vi "AIT 664 - Create Hardware Output Channels Tx Ports.vi"(0 "Device Reference in":T8 format="%.0x", 5 "End System Handle in":u64, 7 "End System References In":T8[](array[typedef]) format="%.0x", 9 "FIFO Index Queues":T13, 11 "error in (no error)":errorcluster) -> (3 "Hardware Output - Tx Ports":T1[](array[typedef]) {"Message Settings"."Transmit Channel Data Reference" format="%.0x"; "Message Settings"."Queue Transmit Channel" format="%.0x"; "Message Settings"."Driver Data"."Num Bits" min=1 max=32; "Message Settings"."Block Data Refs"."Data Reference" format="%.0x"; "Rx Com Udp Port"."Handle" format="%08x"; "Tx Com Udp Port"."Handle" format="%08x"}, 15 "error out":errorcluster)   [LabVIEW 2013, in "AIT 664 Custom Device.lvlib"]
doc: "For each Output VL page, find all of the Tx Mesage Ports Pages and configure the AIT 664 ComUdp port and all of the channels defined by the user for that port.\n\nReturns configured hardware channels and open AIT 664 Com Udp Port."
uses:
  AIT 664 Custom Device.lvlib
  <vilib>/NI Veristand/Custom Device API/Custom Device Item Ref.ctl
  RT Controls/FIFO Index Queues.ctl
  RT Controls/AIT 664 - RT Hardware Channel.ctl
  RT Controls/AIT 664 - RT Message Settings.ctl
  <vilib>/NI Veristand/Custom Device API/Block Data Reference.ctl
  <vilib>/NI Veristand/Custom Device API/Data Reference.ctl
  RT Controls/AIT 664 - Driver Data.ctl
  Controls and Global/Start Bit.ctl
  Controls and Global/Number of Bits.ctl
  <userlib>/ARINC 664/AIT 664 Controls/General/Message Port.ctl
  <userlib>/ARINC 664/AIT 664 Controls/General/Direction.ctl
  <userlib>/ARINC 664/AIT 664 Controls/General/Message Port Type.ctl
  System Explorer/Controls/664 - Sampling Type.ctl
  <vilib>/NI Veristand/Custom Device API/Data Access Type.ctl
  <vilib>/NI Veristand/Custom Device Tools/Custom Device Utility Library/NI VeriStand - Search for All Items by GUID.vi
  Controls and Global/Global.vi
  <vilib>/NI Veristand/Custom Device API/Get Item Property (U32).vi
  <vilib>/NI Veristand/Custom Device API/Get Item Property (Variant).vi
  <instrlib>/AIT 664/Private/AIT 664 Configure/Tx/Open/AIT 664 Tx Open Message Port (ComUdp).vi
  <userlib>/ARINC 664/AIT 664 API.lvlib
  <vilib>/NI Veristand/Custom Device API/Custom Device API.lvlib
  <vilib>/NI Veristand/Custom Device Tools/Custom Device Utility Library/Custom Device Utility Library.lvlib
  <instrlib>/AIT 664/AIT 664.lvlib
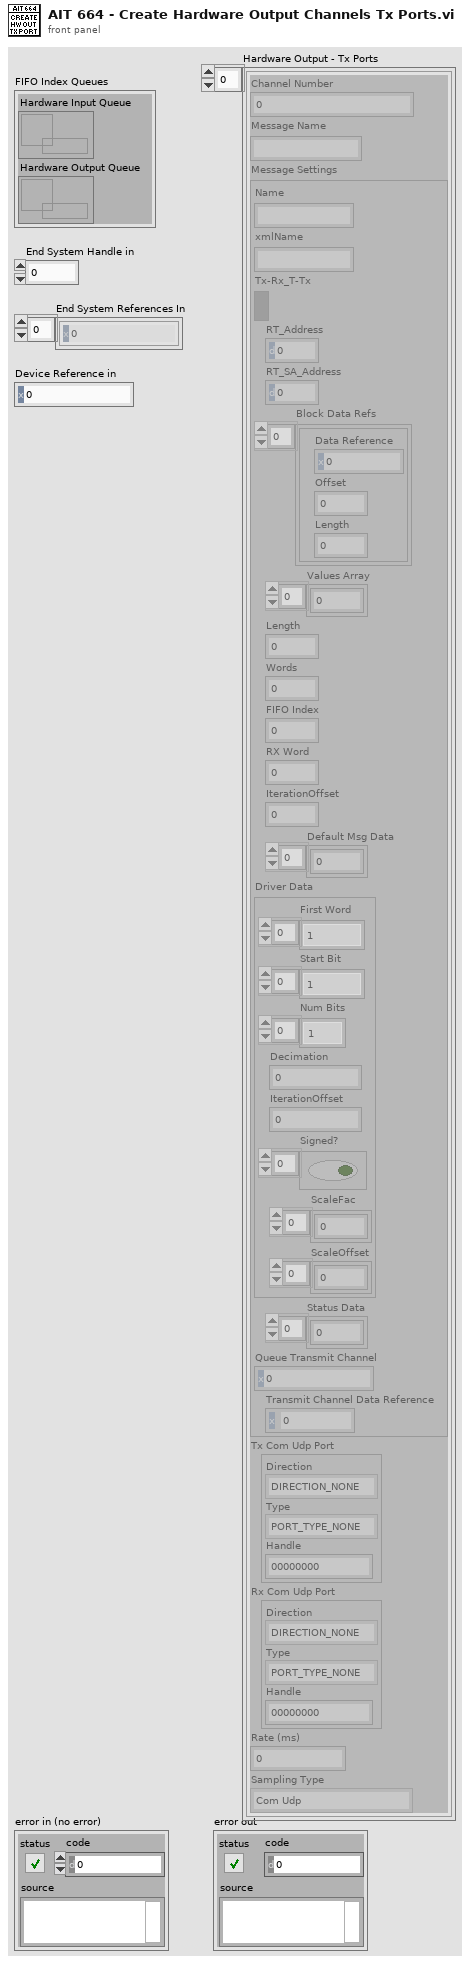
[diagram p1: front panel]
types:
  T1 = typedef "AIT 664 Custom Device.lvlib/AIT 664 - RT Hardware Channel.ctl" = cluster{"Channel Number":u16, "Message Name":string, "Message Settings":T2, "Tx Com Udp Port":T9, "Rx Com Udp Port":T9, "Rate (ms)":u32, "Sampling Type":T12}
  T2 = typedef "AIT 664 Custom Device.lvlib/AIT 664 - RT Message Settings.ctl" = cluster{"Name":string, "xmlName":string, "Tx-Rx_T-Tx":bool, "RT_Address":u8, "RT_SA_Address":u8, "Block Data Refs":T3[], "Values Array":dbl[], "Length":i32, "Words":i32, "FIFO Index":i32, "RX Word":u32, "IterationOffset":i32, "Default Msg Data":u8[], "Driver Data":T5, "Status Data":u32[], "Queue Transmit Channel":T8, "Transmit Channel Data Reference":T4}
  T3 = typedef "Custom Device API.lvlib/Block Data Reference.ctl" = cluster{"Data Reference":T4, "Offset":i32, "Length":i32}
  T4 = typedef "Custom Device API.lvlib/Data Reference.ctl" = i32
  T5 = typedef "AIT 664 Custom Device.lvlib/AIT 664 - Driver Data.ctl" = cluster{"First Word":T6[], "Start Bit":T6[], "Num Bits":T7[], "Decimation":i32, "IterationOffset":i32, "Signed?":bool[], "ScaleFac":dbl[], "ScaleOffset":dbl[]}
  T6 = typedef "AIT 664 Custom Device.lvlib/Start Bit.ctl" = i32
  T7 = typedef "AIT 664 Custom Device.lvlib/Number of Bits.ctl" = i32
  T8 = typedef "Custom Device API.lvlib/Custom Device Item Ref.ctl" = u64
  T9 = typedef "AIT 664 API.lvlib/Message Port.ctl" = cluster{"Direction":T10, "Type":T11, "Handle":u64}
  T10 = typedef "AIT 664 API.lvlib/Direction.ctl" = enum16{"DIRECTION_NONE", "DIRECTION_TX", "DIRECTION_RX"}
  T11 = typedef "AIT 664 API.lvlib/Message Port Type.ctl" = enum16{"PORT_TYPE_NONE", "COM_UDP", "SAP_UDP", "SAP_IP", "SAP_MAC", "COTS_MAC", "COTS_MAC_RAW"}
  T12 = typedef "AIT 664 Custom Device.lvlib/664 - Sampling Type.ctl" = enum16{"Com Udp", "Com Udp Queuing", "Sap Udp", "Sap Ip", "Sap Mac", "Unknown"}
  T13 = typedef "AIT 664 Custom Device.lvlib/FIFO Index Queues.ctl" = cluster{"Hardware Input Queue":refnum<queue>, "Hardware Output Queue":refnum<queue>}
  T14 = typedef "Custom Device API.lvlib/Data Access Type.ctl" = enum16{"Read", "Write"}
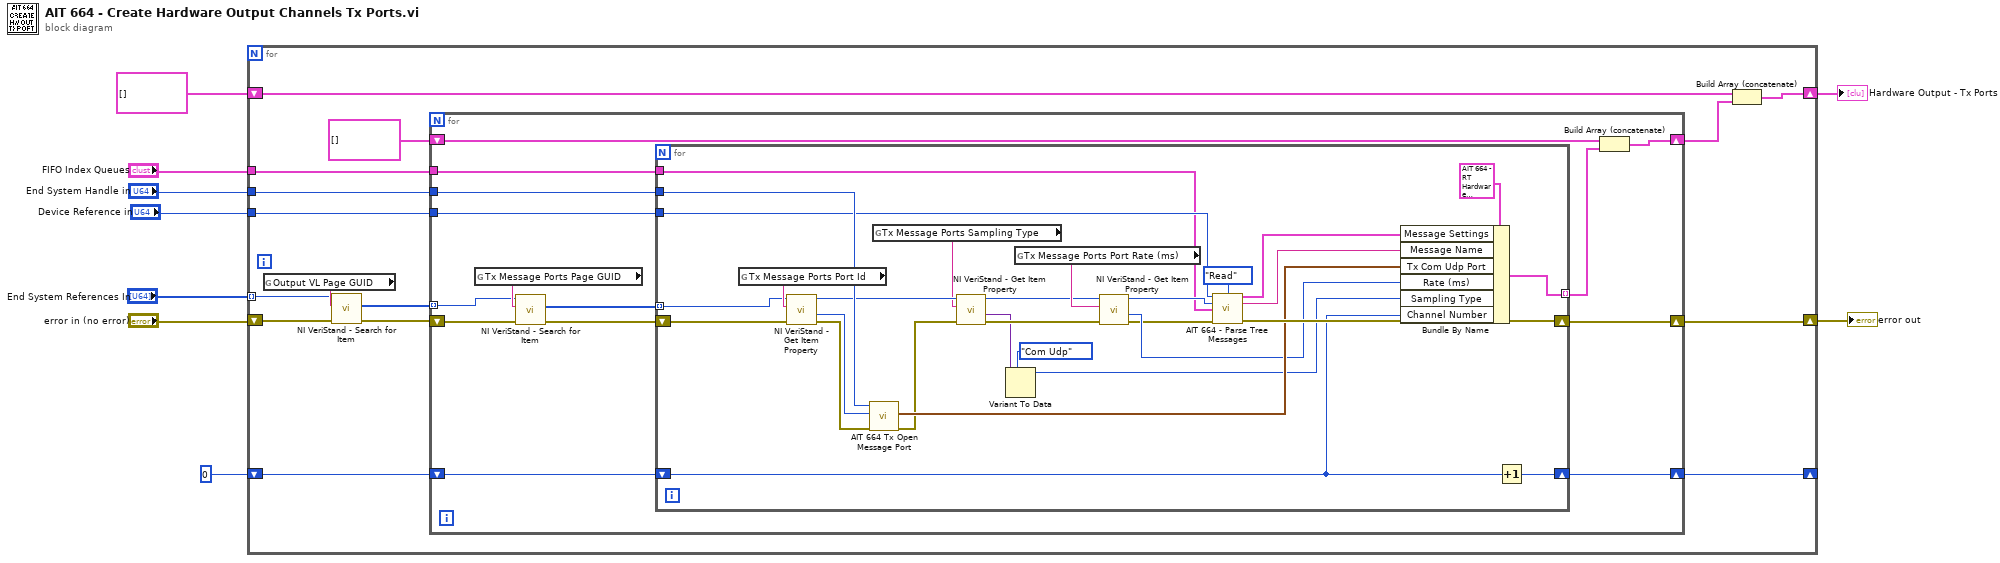
[diagram p0: block diagram]
diagram:
  n1 = for {
    tunnel: "End System References In" -> [w23] mode=indexing
    shift-right: [w19] -> w5
    shift-left: "error in (no error)" -> [w22]
    tunnel: "End System Handle in" -> [w18]
    tunnel: "Device Reference in" -> [w17]
    tunnel: "FIFO Index Queues" -> [w16]
    shift-right: [w12] -> w4
    shift-left: T1[] [] ("element") -> [w13]
    shift-right: [w10] -> _
    shift-left: u16 0 ("Numeric") -> [w11]
    n2 = global read "Global.vi" "Output VL Page GUID"() -> (w24:string)
    n3 = call-poly <vilib>:"NI VeriStand - Search for Item.vi"("error in"=w22, "Item GUID"=w24, "Section Ref in"=w23) -> ("error out"=w21:errorcluster, "Item Refs"=w20:T8[])  [unwired: 5 in, 2 out]
    n4 = for {
      shift-right: [w33] -> w19
      shift-left: w21 -> [w37]
      tunnel: w20 -> [w36] mode=indexing
      tunnel: w18 -> [w32]
      tunnel: w17 -> [w31]
      tunnel: w16 -> [w30]
      shift-right: [w28] -> w14
      shift-left: T1[] [] ("element") -> [w27]
      shift-right: [w25] -> w10
      shift-left: w11 -> [w26]
      n5 = global read "Global.vi" "Tx Message Ports Page GUID"() -> (w38:string)
      n6 = call-poly <vilib>:"NI VeriStand - Search for Item.vi"("error in"=w37, "Item GUID"=w38, "Section Ref in"=w36) -> ("error out"=w35:errorcluster, "Item Refs"=w34:T8[])  [unwired: 5 in, 2 out]
      n7 = for {
        shift-right: [w63] -> w33
        shift-left: w35 -> [w66]
        tunnel: w34 -> [w65] mode=indexing
        tunnel: w32 -> [w62]
        tunnel: w31 -> [w42]
        tunnel: w30 -> [w39]
        tunnel: [w56] -> w29 mode=indexing
        shift-right: [w47] -> w25
        shift-left: w26 -> [w46]
        n8 = global read "Global.vi" "Tx Message Ports Port Id"() -> (w67:string)
        n9 = call-poly <vilib>:"NI VeriStand - Get Item Property.vi"("error in (no error)"=w66, "Property Name"=w67, "Item Ref in"=w65) -> ("error out"=w60:errorcluster, "Value"=w61:u32, "Item Ref out"=w54:T8)  [unwired: 5 in, 1 out]
        n10 = call-poly <instrlib>:"AIT 664 Tx Open Message Port.vi"("error in"=w60, "Port Id in"=w61, "End System Handle in"=w62) -> ("error out"=w51:errorcluster, "Tx Com Udp Port out"=w57:T9)  [unwired: 4 in, 1 out]
        n11 = global read "Global.vi" "Tx Message Ports Sampling Type"() -> (w50:string)
        n12 = call-poly <vilib>:"NI VeriStand - Get Item Property.vi"("error in (no error)"=w51, "Property Name"=w50, "Item Ref in"=w54) -> ("error out"=w52:errorcluster, "Value"=w48:variant, "Item Ref out"=w53:T8)  [unwired: 5 in, 1 out]
        n13 = Variant To Data(type=664_-_Sampling_Type."Com Udp" ("Sampling Type"), Variant=w48) -> (data=w41:T12)  [unwired: 1 in, 1 out]
        n14 = global read "Global.vi" "Tx Message Ports Port Rate (ms)"() -> (w64:string)
        n15 = call-poly <vilib>:"NI VeriStand - Get Item Property.vi"("error in (no error)"=w52, "Property Name"=w64, "Item Ref in"=w53) -> ("error out"=w44:errorcluster, "Value"=w55:u32, "Item Ref out"=w43:T8)  [unwired: 5 in, 1 out]
        n16 = call "AIT 664 - Parse Tree Messages.vi"("Device Reference in"=w42, "Access Type"=Data_Access_Type."Read", "Message Reference in"=w43, "FIFO Index Queues in"=w39, "error in"=w44) -> ("Message Settings out"=w59:T2, "Message Name out"=w58:string, "error out"=w63:errorcluster)  [unwired: 8 in]
        n17 = Bundle By Name(cluster=T1 {"Channel Number"=0, "Message Name"="", "Message Settings"={"Name"="", "xmlName"="", "Tx-Rx_T-Tx"=FALSE, "RT_Address"=0, "RT_SA_Address"=0, "Block Data Refs"=[], "Values Array"=[], "Length"=0, "Words"=0, "FIFO Index"=0, "RX Word"=0, "IterationOffset"=0, "Default Msg Data"=[], "Driver Data"={"First Word"=[], "Start Bit"=[], "Num Bits"=[], "Decimation"=0, "IterationOffset"=0, "Signed?"=[], "ScaleFac"=[], "ScaleOffset"=[]}, "Status Data"=[], "Queue Transmit Channel"=0, "Transmit Channel Data Reference"=0}, "Tx Com Udp Port"={"Direction"=enum."DIRECTION_NONE", "Type"=enum."PORT_TYPE_NONE", "Handle"=0}, "Rx Com Udp Port"={"Direction"=enum."DIRECTION_NONE", "Type"=enum."PORT_TYPE_NONE", "Handle"=0}, "Rate (ms)"=0, "Sampling Type"=enum."Com Udp"} ("Hardware Channel"), "Message Settings"=w59, "Message Name"=w58, "Tx Com Udp Port"=w57, "Rate (ms)"=w55, "Sampling Type"=w41, "Channel Number"=w46) -> (w56:T1)
        n18 = Increment(x=w46) -> (x+1=w47:u16)
      }
      n19 = Build Array (concatenate)(w27, w29) -> (w28:T1[])
    }
    n20 = Build Array (concatenate)(w13, w14) -> (w12:T1[])
  }
  "error out" <- w5
  "Hardware Output - Tx Ports" <- w4
